vi "pre-processamento.vi"() -> ()   [LabVIEW 2024]
uses:
  <vilib>/numeric/Random Number (Range) DBL.vi
panel:
  out "fator de potência 3":dbl
  out "Potencia \nativa C":string[][](table)
  out "Tensão e Corrent C":string[][](table)
  out "Waveform Graph 3":dbl[](graph) caption="Potência Ativa C"
  out "fator de potência 2":dbl
  out "Potencia \nativa B":string[][](table)
  out "Tensão e Corrent B":string[][](table)
  out "Waveform Graph 2":dbl[](graph) caption="Potência Ativa B"
  out "fator de potência":dbl
  out "Potencia \nativa":string[][](table)
  out "Tensão e Corrent A":string[][](table)
  out "Waveform Graph":dbl[](graph) caption="Potência Ativa A"
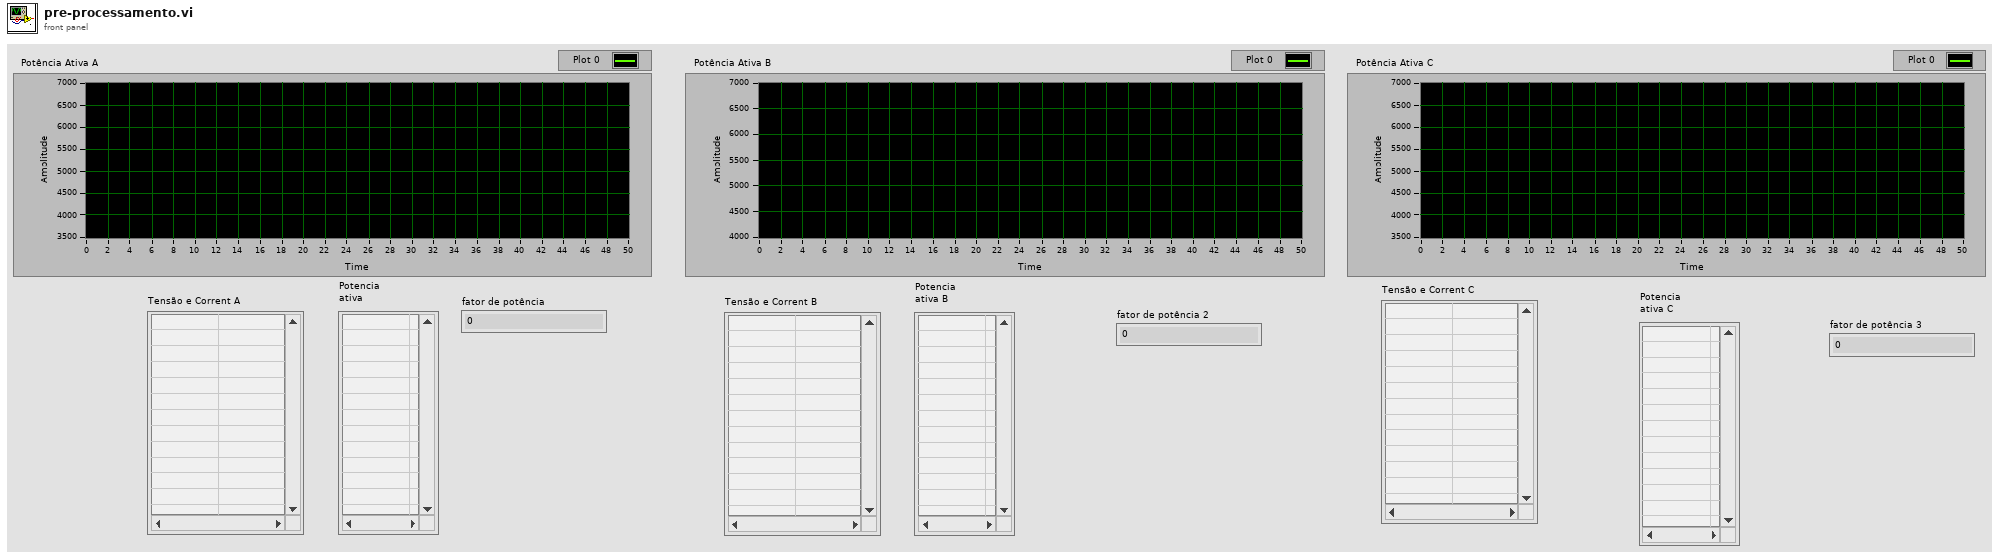
[diagram p1: front panel]
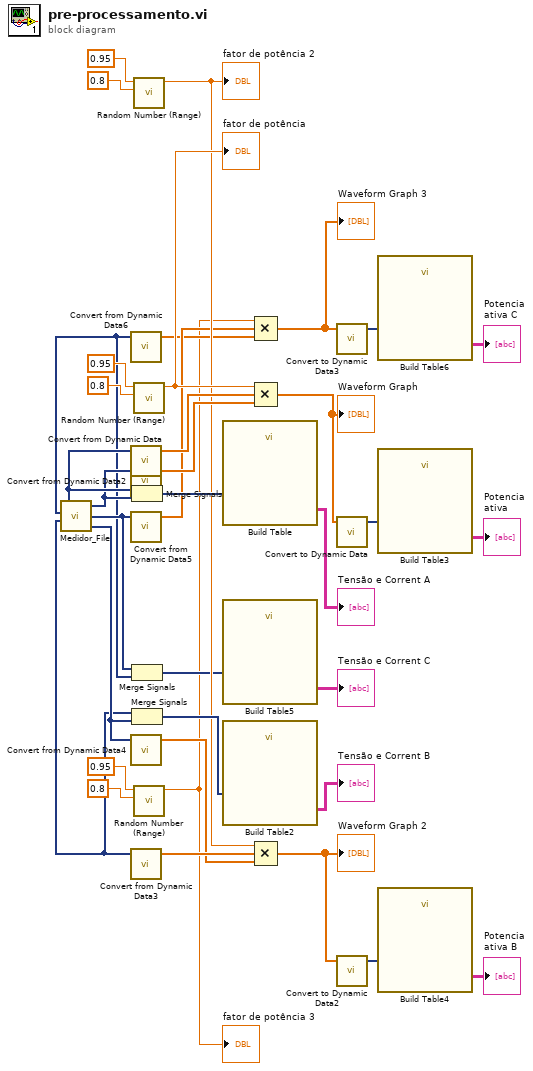
[diagram p0: block diagram]
diagram:
  n1 = call "Medidor_File.vi"() -> ("Corrente Fase C"=w14:dynamicdata, "Corrente Fase B"=w2:dynamicdata, "Corrente Fase A"=w29:dynamicdata, "Tensão Fase C"=w13:dynamicdata, "Tensão Fase B"=w1:dynamicdata, "Tensão Fase A"=w30:dynamicdata)  [unwired: 1 out]
  n2 = call "Convert from Dynamic Data6"("Dynamic Data Type"=w1) -> ("Array"=w11:dbl[])  [unwired: 3 in]
  n3 = call "Convert from Dynamic Data"("Dynamic Data Type"=w30) -> ("Array"=w36:dbl[])  [unwired: 3 in]
  n4 = call "Convert from Dynamic Data2"("Dynamic Data Type"=w29) -> ("Array"=w35:dbl[])  [unwired: 3 in]
  n5 = call "Convert from Dynamic Data5"("Dynamic Data Type"=w2) -> ("Array"=w12:dbl[])  [unwired: 3 in]
  n6 = call "Convert from Dynamic Data4"("Dynamic Data Type"=w14) -> ("Array"=w23:dbl[])  [unwired: 3 in]
  n7 = call "Convert from Dynamic Data3"("Dynamic Data Type"=w13) -> ("Array"=w24:dbl[])  [unwired: 3 in]
  n8 = Merge Signals(w30, w29) -> (w28:dynamicdata)
  n9 = Merge Signals(w2, w1) -> (w6:dynamicdata)
  n10 = Merge Signals(w13, w14) -> (w18:dynamicdata)
  n11 = call-poly <vilib>:"Random Number (Range).vi"("lower bound (0)"=0.8, "upper bound (100)"=0.95) -> ("number"=w15:dbl)  [unwired: 9 in]
  "fator de potência 2" <- w15
  n12 = call-poly <vilib>:"Random Number (Range).vi"("lower bound (0)"=0.8, "upper bound (100)"=0.95) -> ("number"=w25:dbl)  [unwired: 9 in]
  "fator de potência" <- w25
  n13 = call-poly <vilib>:"Random Number (Range).vi"("lower bound (0)"=0.8, "upper bound (100)"=0.95) -> ("number"=w3:dbl)  [unwired: 9 in]
  "fator de potência 3" <- w3
  n14 = call "Build Table"("Signals"=w28) -> ("Table"=→"Tensão e Corrent A":string[][])  [unwired: 4 in, 6 out]
  n15 = call "Build Table5"("Signals"=w6) -> ("Table"=→"Tensão e Corrent C":string[][])  [unwired: 4 in, 6 out]
  n16 = call "Build Table2"("Signals"=w18) -> ("Table"=→"Tensão e Corrent B":string[][])  [unwired: 4 in, 6 out]
  n17 = Compound Arithmetic op=MULTIPLY(w3, w12, w11) -> (w8:dbl[])
  "Waveform Graph 3" <- w8
  n18 = Compound Arithmetic op=MULTIPLY(w25, w36, w35) -> (w32:dbl[])
  "Waveform Graph" <- w32
  n19 = Compound Arithmetic op=MULTIPLY(w15, w24, w23) -> (w20:dbl[])
  "Waveform Graph 2" <- w20
  n20 = call "Convert to Dynamic Data3"("Array"=w8) -> ("Dynamic Data Type"=w7:dynamicdata)  [unwired: 3 in]
  n21 = call "Convert to Dynamic Data"("Array"=w32) -> ("Dynamic Data Type"=w31:dynamicdata)  [unwired: 3 in]
  n22 = call "Convert to Dynamic Data2"("Array"=w20) -> ("Dynamic Data Type"=w19:dynamicdata)  [unwired: 3 in]
  n23 = call "Build Table6"("Signals"=w7) -> ("Table"=→"Potencia \nativa C":string[][])  [unwired: 4 in, 6 out]
  n24 = call "Build Table3"("Signals"=w31) -> ("Table"=→"Potencia \nativa":string[][])  [unwired: 4 in, 6 out]
  n25 = call "Build Table4"("Signals"=w19) -> ("Table"=→"Potencia \nativa B":string[][])  [unwired: 4 in, 6 out]
